vi "Read Setpoint.vi"(7 "Channel (0: Channel A)":u16(ring) items=["Channel A", "Channel B"], 8 "error in (no error)":errorcluster, 11 "BH Druck PACE Series in":refnum<class "BH Druck PACE Series.lvclass">) -> (0 "error out":errorcluster, 2 "Setpoint":dbl format="%#.10g", 3 "BH Druck PACE Series out":refnum<class "BH Druck PACE Series.lvclass">)   [LabVIEW 2022 SP3, in "BH Druck PACE Series.lvclass"]
uses:
  BH Druck PACE Series.lvclass
  BH Druck PACE Series.lvclass/BH Druck PACE Series.ctl
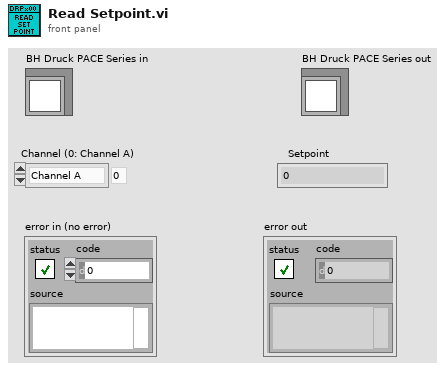
[diagram p1: front panel]
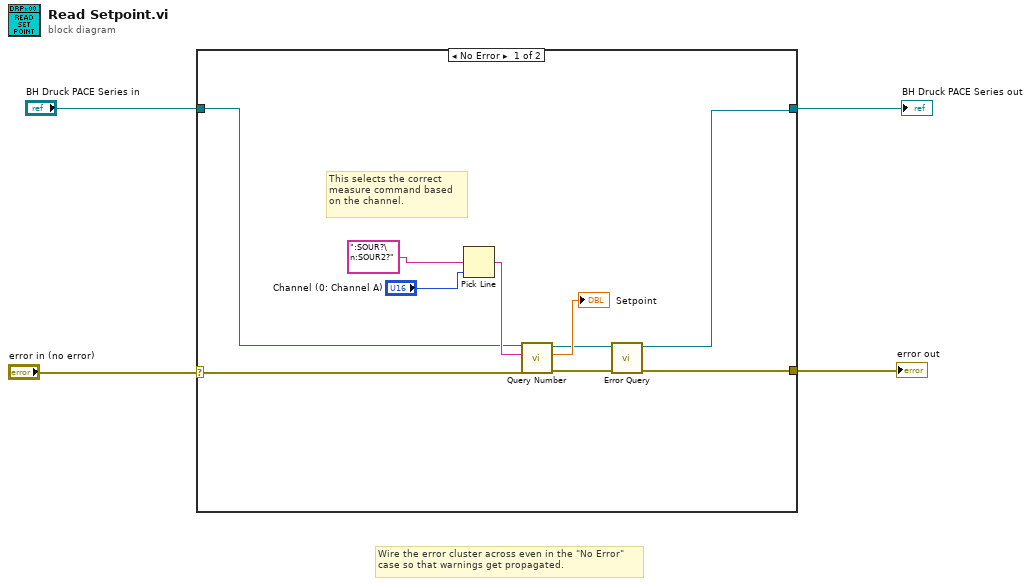
[diagram p0: block diagram]
diagram:
  # "Wire the error cluster across even in the \"No Error\"\ncase so that warnings get propagated."
  n1 = case shown="No Error" "error in (no error)" {
    selector: "error in (no error)" -> [w8 w16]
    tunnel: [w7 w16] -> w3
    tunnel: [w5 w15] -> w1
    tunnel: "BH Druck PACE Series in" -> [w6 w15]
    frame No Error {
      # "This selects the correct\nmeasure command based\non the channel."
      n2 = Pick Line(multi-line string=":SOUR?\n:SOUR2?", line index="Channel (0: Channel A)") -> (output string=w13:string)  [unwired: 1 in]
      n3 = call-dynamic "Query Number.vi"("error in (no error)"=w8, "Query String"=w13, "BH Druck PACE Series in"=w6) -> ("error out"=w14:errorcluster, "Numeric Result"=→"Setpoint":dbl, "BH Druck PACE Series out"=w11:refnum<class "BH Druck PACE Series.lvclass">)  [unwired: 6 in]
      n4 = call-dynamic "Error Query.vi"("error in (no error)"=w14, "BH Druck PACE Series in"=w11) -> ("error out"=w7:errorcluster, "BH Druck PACE Series out"=w5:refnum<class "BH Druck PACE Series.lvclass">)  [unwired: 8 in]
    }
    frame Error {
    }
  }
  "error out" <- w3
  "BH Druck PACE Series out" <- w1
